vi "tdsget.vi"(1 "VISA Port In":refnum<visa-resource-name>, 7 "Channel Number":u16=1 min=1 max=2 step=1, 9 "ps/point":u32, 11 "ns/div":u32, 12 "Error In (No Error)":errorcluster) -> (3 "VISA Port Out":refnum<visa-resource-name>, 8 "TDS Data":u16[](array[numeric]), 14 "Error Out":errorcluster)   [LabVIEW 2009]
panel:
  out "Numeric":i32
  out "read buffer":string
  in  "Required TDS Data Type":u16[](array[numeric])
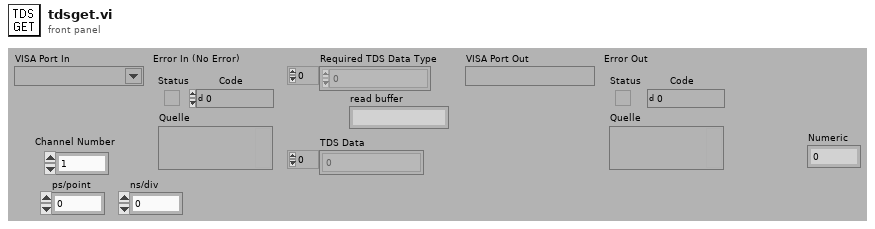
[diagram p1: front panel]
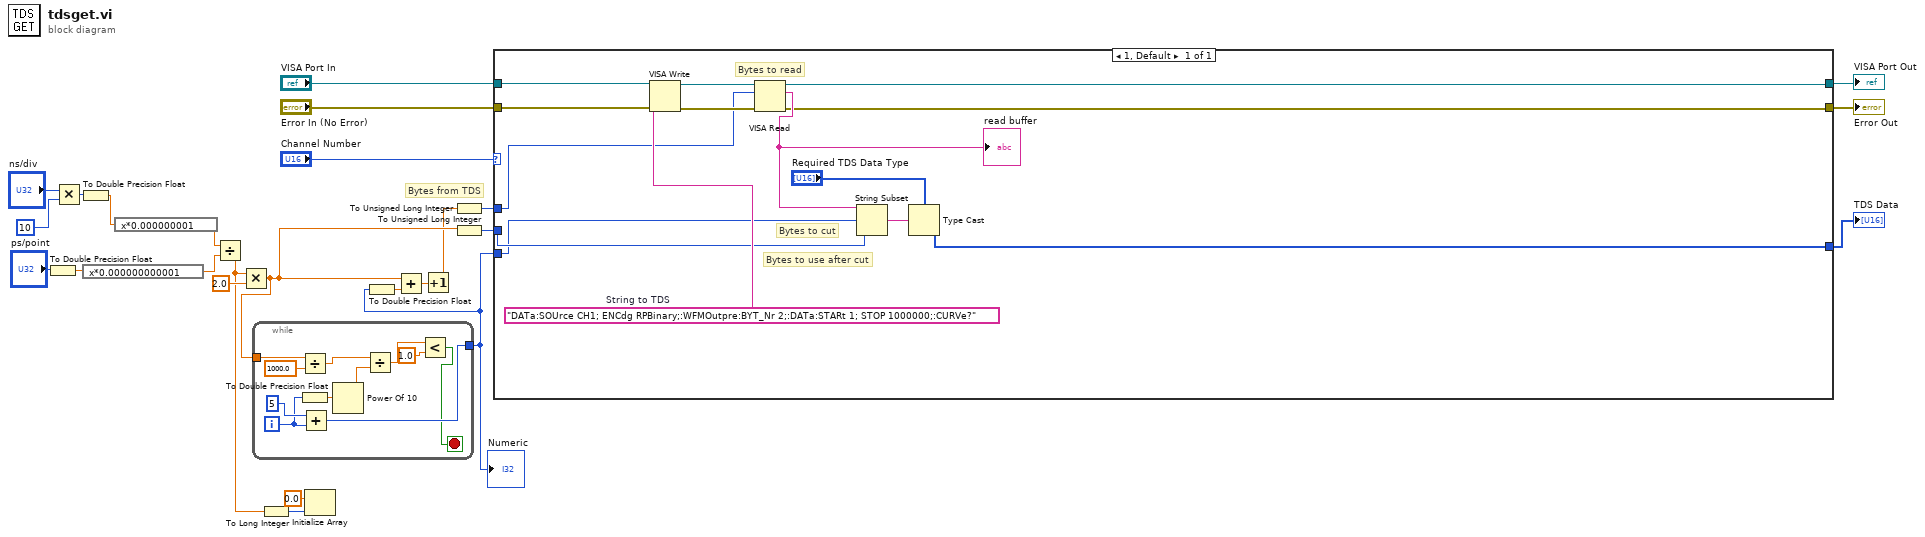
[diagram p0: block diagram]
diagram:
  # "Bytes from TDS"
  n1 = To Double Precision Float(number="ps/point") -> (double precision float=w15:dbl)
  n2 = Multiply(x="ns/div", y=u32 10) -> (x*y=w17:u32)
  n3 = To Double Precision Float(number=w17) -> (double precision float=w14:dbl)
  n4 = expression code="x*0.000000000001"(w15) -> (w12:dbl)
  n5 = expression code="x*0.000000001"(w14) -> (w13:dbl)
  n6 = Divide(x=w13, y=w12) -> (x/y=w7:dbl)
  n7 = Multiply(x=w7, y=2.0) -> (x*y=w5:dbl)
  n8 = while {
    tunnel: w5 -> [w32]
    tunnel: [w35] -> w3
    i -> [w34]
    stop <- w26 stop-if-true
    n9 = Divide(x=w32, y=1000.0) -> (x/y=w28:dbl)
    n10 = To Double Precision Float(number=w34) -> (double precision float=w33:dbl)
    n11 = Add(x=5, y=w34) -> (x+y=w35:i32)
    n12 = Power Of 10(x=w33) -> (10^x=w29:dbl)
    n13 = Divide(x=w28, y=w29) -> (x/y=w27:dbl)
    n14 = Less?(x=w27, y=1.0) -> (x < y?=w26:bool)
  }
  "Numeric" <- w3
  n15 = To Long Integer(number=w7) -> (32bit integer=w8:i32)
  n16 = Initialize Array(0.0 ("element"), w8) -> ()  [unwired: 1 out]
  n17 = To Double Precision Float(number=w3) -> (double precision float=w4:dbl)
  n18 = Add(x=w5, y=w4) -> (x+y=w2:dbl)
  n19 = Increment(x=w2) -> (x+1=w1:dbl)
  n20 = To Unsigned Long Integer(number=w1) -> (unsigned 32bit integer=w10:u32)
  n21 = To Unsigned Long Integer(number=w5) -> (unsigned 32bit integer=w9:u32)
  n22 = case shown="1, Default" "Channel Number" {
    tunnel: [w41] -> w25
    tunnel: "Error In (No Error)" -> [w50]
    tunnel: "VISA Port In" -> [w49]
    tunnel: [w42] -> w22
    tunnel: [w40] -> w21
    tunnel: w10 -> [w39]
    tunnel: w9 -> [w38]
    tunnel: w3 -> [w37]
    frame 1, Default {
      w48 = "DATa:SOUrce CH1; ENCdg RPBinary;:WFMOutpre:BYT_Nr 2;:DATa:STARt 1; STOP 1000000;:CURVe?"  # String to TDS
      # "Bytes to use after cut"
      # "Bytes to cut"
      # "Bytes to read"
      n23 = VISA Write(VISA resource name=w49, write buffer=w48, error in (no error)=w50) -> (VISA resource name out=w45:refnum<visa-resource-name>, error out=w44:errorcluster)  [unwired: 1 out]
      n24 = VISA Read(VISA resource name=w45, byte count=w39, error in (no error)=w44) -> (VISA resource name out=w41:refnum<visa-resource-name>, read buffer=w43:string, error out=w40:errorcluster)  [unwired: 1 out]
      "read buffer" <- w43
      n25 = String Subset(string=w43, offset (0)=w37, length (rest)=w38) -> (substring=w46:string)
      n26 = Type Cast(type="Required TDS Data Type", x=w46) -> (*(type *) &x=w42:u16[])
    }
  }
  "Error Out" <- w21
  "VISA Port Out" <- w25
  "TDS Data" <- w22
